vi "Build Order.vi"(8 "error in (no error)":errorcluster, 9 "Name":string, 10 "Customer":refnum<class "Message Enqueuer.lvclass">, 11 "Order":cluster{"Drink type":T1, "Options":T2[]}[](array[cluster])) -> (0 "error out":errorcluster, 2 "Cost":dbl, 3 "Order Out":refnum<class "Order.lvclass">)   [LabVIEW 2023, in "Order.lvclass"]
doc: "Generate and initialize an Order object."
uses:
  Classes/Order/Order.lvclass
  Classes/Beverages/TypeDefs/Drink Type.ctl
  Classes/Beverages/TypeDefs/Options.ctl
  <vilib>/ActorFramework/Message Enqueuer/Message Enqueuer.lvclass
  Classes/Beverages/Beverage/Beverage.lvclass
  Classes/Beverages/Beverage/Beverage.lvclass/Beverage.ctl
  Classes/Order/Order.lvclass/Order.ctl
  Classes/Beverages/Beverage/Write Drink Type.vi
  Classes/Beverages/Beverage/Write Options.vi
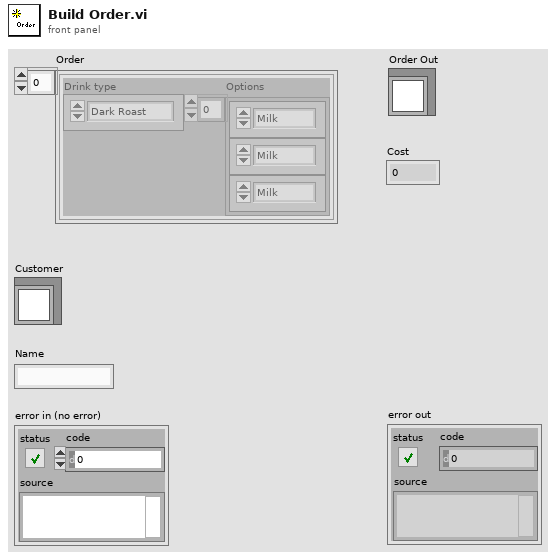
[diagram p1: front panel]
types:
  T1 = typedef "Beverage.lvclass/Drink Type.ctl" = enum16{"Dark Roast", "Decaf", "Espresso", "House Blend"}
  T2 = typedef "Beverage.lvclass/Options.ctl" = enum16{"<None>", "Milk", "Mocha", "Soy", "Whip"}
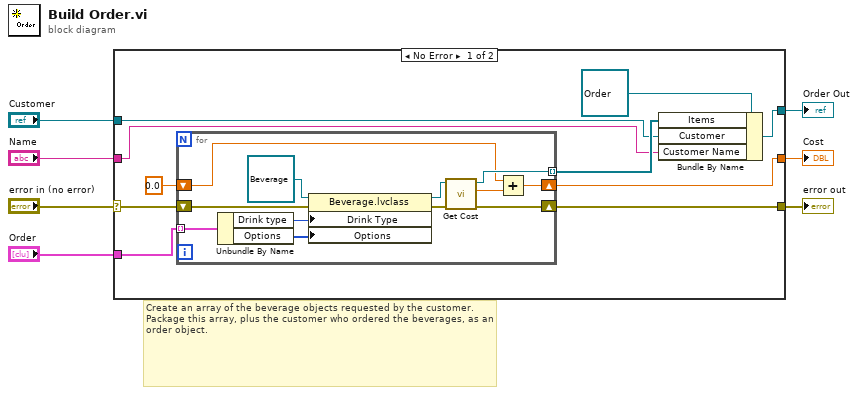
[diagram p0: block diagram]
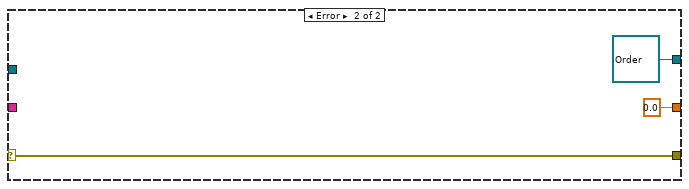
[diagram p2: hidden frame]
diagram:
  # "Create an array of the beverage objects requested by the customer.  Package this array, plus the customer who ordered the beverages, as an order object."
  n1 = case shown="No Error" "error in (no error)" {
    selector: "error in (no error)" -> [w10 w32]
    tunnel: "Order" -> [w17 _]
    tunnel: [w14 refnum<class "Order.lvclass"> refnum ("Order.lvclass")] -> w6
    tunnel: "Customer" -> [w13 _]
    tunnel: [w9 w32] -> w3
    tunnel: [w12 0.0] -> w2
    tunnel: "Name" -> [w8 _]
    frame No Error {
      n2 = for {
        tunnel: w17 -> [w29] mode=indexing
        tunnel: [w28] -> w15 mode=indexing
        shift-right: [w27] -> w12
        shift-left: 0.0 -> [w25]
        shift-right: [w18] -> w9
        shift-left: w10 -> [w19]
        n3 = Unbundle By Name(w29) -> ("Drink type"=w23:T1, "Options"=w22:T2[])
        n4 = property on="Property Node" class="Beverage.lvclass"(reference=refnum<class "Beverage.lvclass"> refnum ("Beverage in"), error in=w19, "Drink Type"=w23, "Options"=w22) -> (reference out=w21:refnum<class "Beverage.lvclass">, error out=w20:errorcluster)
        n5 = call "Get Cost.vi"("error in (no error)"=w20, "Beverage in"=w21) -> ("error out"=w18:errorcluster, "Cost"=w26:dbl, "Beverage out"=w28:refnum<class "Beverage.lvclass">)  [unwired: 7 in]
        n6 = Add(x=w25, y=w26) -> (x+y=w27:dbl)
      }
      n7 = Bundle By Name(cluster=refnum<class "Order.lvclass"> refnum ("Order.lvclass"), "Items"=w15, "Customer"=w13, "Customer Name"=w8) -> (w14:refnum<class "Order.lvclass">)
    }
    frame Error {
    }
  }
  "Order Out" <- w6
  "error out" <- w3
  "Cost" <- w2
